vi "test_fpga_motor_dir.vi"() -> ()   [LabVIEW 2018]
panel:
  in  "stop":bool
  out "x .and. y? 2":bool
  out "x .and. y?":bool
  in  "Slide":i16(slide) scale=-2000.0..2000.0
  in  "limit":i16
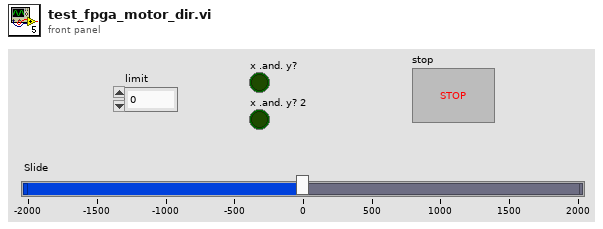
[diagram p1: front panel]
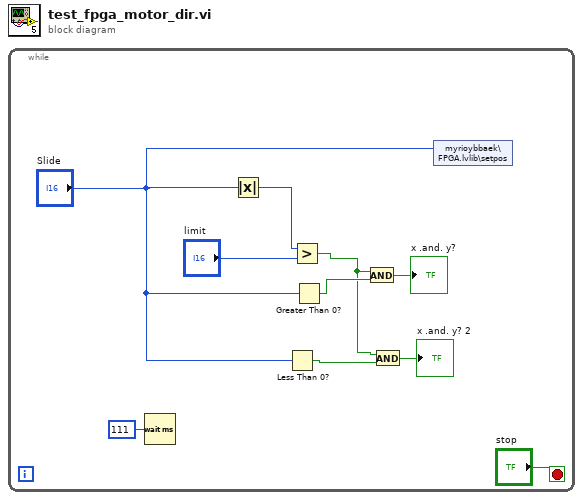
[diagram p0: block diagram]
diagram:
  n1 = while {
    stop <- "stop" stop-if-true
    n2 = Wait (ms)(milliseconds to wait=u32 111) -> ()  [unwired: 1 out]
    n3 = Absolute Value(x="Slide") -> (abs(x)=w9:i16)
    n4 = Less Than 0?(x="Slide") -> (x < 0?=w6:bool)
    n5 = Greater?(x=w9, y="limit") -> (0:w5:bool)
    n6 = Greater Than 0?(x="Slide") -> (x > 0?=w8:bool)
    n7 = And(x=w5, y=w8) -> (x .and. y?=→"x .and. y?":bool)
    n8 = And(x=w5, y=w6) -> (x .and. y?=→"x .and. y? 2":bool)
    n9 = shared-variable "myrioybbaek\\FPGA.lvlib\\setpos"("Slide") -> ()  [unwired: 1 in, 1 out]
  }
